vi "VRM Calculate Sweep Rates.vi"(8 "error in (no error)":errorcluster, 9 "Sweep rate (T/min)":dbl, 10 "Target Field (T)":dbl[](array[numeric]), 11 "Initial Field (T)":dbl[](array[numeric])) -> (0 "error out":errorcluster, 1 "time (min)":dbl, 3 "Sweep Rate Field (T/min)":dbl[](array[numeric]))   [LabVIEW 2016, in "Instrument.OxfordVRM.lvclass"]
uses:
  Instrument.OxfordVRM.lvclass
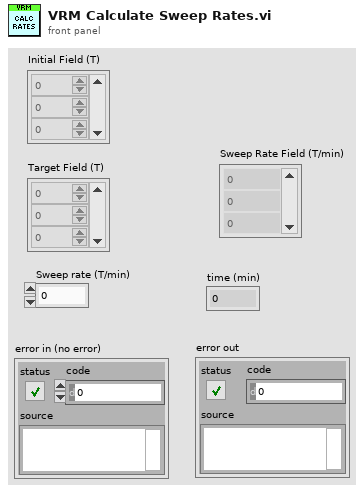
[diagram p1: front panel]
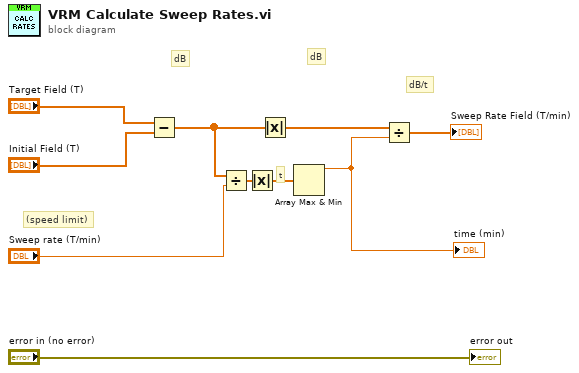
[diagram p0: block diagram]
diagram:
  # "dB/t"
  # "dB"
  # "(speed limit)"
  # "t"
  # "dB"
  n1 = Subtract(x="Target Field (T)", y="Initial Field (T)") -> (x-y=w4:dbl[])
  n2 = Divide(x=w4, y="Sweep rate (T/min)") -> (x/y=w9:dbl[])
  n3 = Absolute Value(x=w9) -> (abs(x)=w6:dbl[])
  n4 = Absolute Value(x=w4) -> (abs(x)=w5:dbl[])
  n5 = Array Max & Min(array=w6) -> (max value=w8:dbl)  [unwired: 3 out]
  "time (min)" <- w8
  n6 = Divide(x=w5, y=w8) -> (x/y=→"Sweep Rate Field (T/min)":dbl[])
  "error out" <- "error in (no error)"
